vi "getImageFromBuffer.vi"(8 "error in (no error)":errorcluster, 9 "String":string, 10 "ImageBufferRef":refnum<k7>, 11 "ICCameraAcquisitor in":refnum<class "ICCameraAcquisitor.lvclass">) -> (0 "error out":errorcluster, 2 "ImageBufferRef out":refnum<k7>, 3 "ICCameraAcquisitor out":refnum<class "ICCameraAcquisitor.lvclass">)   [LabVIEW 2009, in "Hardware.lvlib" / "Channels.lvlib" / "ICCameraAcquisitor.lvclass"]
uses:
  ICCameraAcquisitor.lvclass
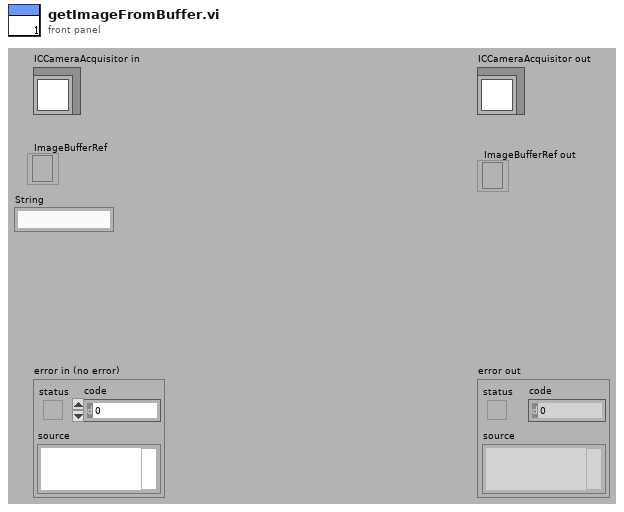
[diagram p1: front panel]
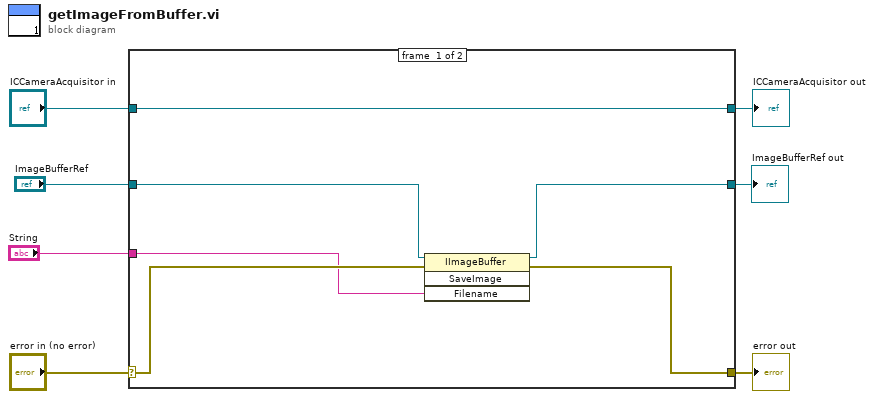
[diagram p0: block diagram]
diagram:
  n1 = case shown="No Error" "error in (no error)" {
    selector: "error in (no error)" -> [w11 w15]
    tunnel: [w10 w15] -> w6
    tunnel: [w13 w14] -> w4
    tunnel: "ICCameraAcquisitor in" -> [w13 w14]
    tunnel: "ImageBufferRef" -> [w12 _]
    tunnel: [w9 _] -> w2
    tunnel: "String" -> [w8 _]
    frame #0 {
      n2 = invoke class="IImageBuffer" method="SaveImage"(reference=w12, error in=w11, "Filename"=w8) -> (reference out=w9:refnum<k7>, error out=w10:errorcluster)  [unwired: 1 in, 2 out]
    }
    frame #1 {
    }
  }
  "error out" <- w6
  "ICCameraAcquisitor out" <- w4
  "ImageBufferRef out" <- w2
